vi "init subpanel.vi"(0 "References in":T2, 5 "Sub Panel":refnum<vi>, 7 "VI refnum":refnum<vi>, 9 "node ref":T1, 11 "error in (no error)":errorcluster) -> (15 "error IO":errorcluster)   [LabVIEW 2013, in "Scaling editor node.lvclass"]
uses:
  Scaling editor node.lvclass
  <vilib>/NI/DCAF Table API/Table Manager/references.ctl
  <vilib>/NI/Configuration Framework/Node/StopEvent.ctl
  <vilib>/NI/Configuration Framework/Node/RefreshUIEvent.ctl
  <vilib>/NI/Configuration Framework/Node/CacheState.ctl
  <vilib>/NI/Configuration Framework/Node/NodeChangeEvent.ctl
  <vilib>/NI/Configuration Framework/Node/NodeRef.ctl
  <vilib>/NI/Configuration Framework/Node/NISE_CEF_Node.lvclass
  <vilib>/NI/DCAF/Tag Editor Core/control module/editor node/channel action event.ctl
  <vilib>/NI/DCAF/Tag Editor Core/control module/editor node/dialog output action.ctl
  <vilib>/NI/Tag Bus Module Framework/channel/TBM channel.lvclass
  <vilib>/NI/Tag Bus/tag/tag descriptor.lvclass
  <vilib>/NI/AMC/Message Queue.ctl
  <vilib>/NI/AMC/Message.ctl
  <vilib>/NI/Tools/Keyed Array/KeyedArray.ctl
  <vilib>/NI/Configuration Framework/Node/UserEventRef.ctl
  <vilib>/NI/Configuration Framework/Controls/EventCluster.ctl
  <vilib>/NI/DCAF/Tag Editor Core/control module/editor node/control module editor.lvclass
  <vilib>/NI/Tools/Keyed Array/Tools_KeyedArray.lvlib
  <vilib>/NI/AMC/AMC.lvlib
  <vilib>/NI/Configuration Framework/NISE_CEF_TreeControl.lvlib
  <vilib>/NI/DCAF Table API/Table Manager/Table Manager.lvclass
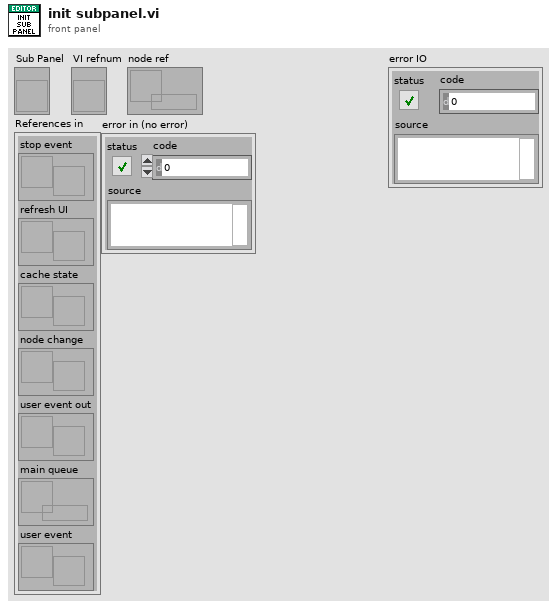
[diagram p1: front panel]
types:
  T1 = typedef "NISE_CEF_Node.lvclass/NodeRef.ctl" = refnum<data-value>
  T2 = typedef "Table Manager.lvlib/Table Manager.lvclass/references.ctl" = cluster{"stop event":T3, "refresh UI":T4, "cache state":T5, "node change":T6, "user event out":refnum<user-event>, "main queue":T7, "user event":T8}
  T3 = typedef "NISE_CEF_Node.lvclass/StopEvent.ctl" = refnum<user-event>
  T4 = typedef "NISE_CEF_Node.lvclass/RefreshUIEvent.ctl" = refnum<user-event>
  T5 = typedef "NISE_CEF_Node.lvclass/CacheState.ctl" = refnum<user-event>
  T6 = typedef "NISE_CEF_Node.lvclass/NodeChangeEvent.ctl" = refnum<user-event>
  T7 = typedef "AMC.lvlib/Message Queue.ctl" = refnum<queue>
  T8 = typedef "NISE_CEF_Node.lvclass/UserEventRef.ctl" = refnum<user-event>
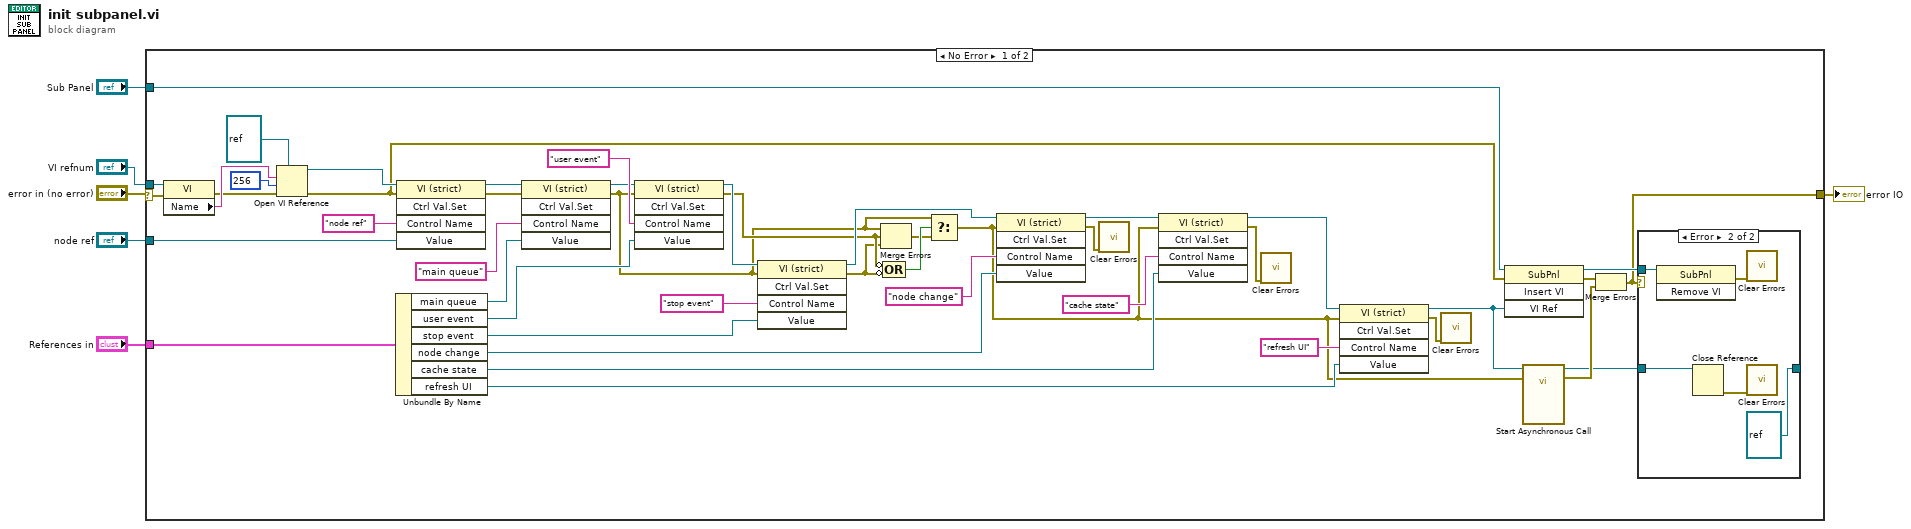
[diagram p0: block diagram]
diagram:
  n1 = case shown="No Error" "error in (no error)" {
    selector: "error in (no error)" -> [w8 w59]
    tunnel: "VI refnum" -> [w48 _]
    tunnel: "References in" -> [w44 _]
    tunnel: "Sub Panel" -> [w18 _]
    tunnel: "node ref" -> [w9 _]
    tunnel: [w7 w59] -> w1
    frame No Error {
      n2 = property class="VI"(reference=w48, error in=w8) -> (error out=w49:errorcluster, "Name"=w50:string)  [unwired: 1 out]
      n3 = Open VI Reference(type specifier VI Refnum (for type only)=refnum<vi> refnum, vi path=w50, options=256, error in (no error)=w49) -> (vi reference=w46:refnum<vi>, error out=w17:errorcluster)  [unwired: 2 in]
      n4 = Unbundle By Name(w44) -> ("main queue"=w32:T7, "user event"=w43:T8, "stop event"=w40:T3, "node change"=w38:T6, "cache state"=w23:T5, "refresh UI"=w19:T4)
      n5 = invoke class="VI (strict)" method="Ctrl Val.Set"(reference=w46, error in=w17, "Control Name"="node ref", "Value"=w9) -> (reference out=w34:refnum<vi>, error out=w33:errorcluster)  [unwired: 1 in, 3 out]
      n6 = invoke class="VI (strict)" method="Ctrl Val.Set"(reference=w34, error in=w33, "Control Name"="main queue", "Value"=w32) -> (reference out=w31:refnum<vi>, error out=w27:errorcluster)  [unwired: 1 in, 3 out]
      n7 = invoke class="VI (strict)" method="Ctrl Val.Set"(reference=w31, error in=w27, "Control Name"="user event", "Value"=w43) -> (reference out=w41:refnum<vi>, error out=w30:errorcluster)  [unwired: 1 in, 3 out]
      n8 = invoke class="VI (strict)" method="Ctrl Val.Set"(reference=w41, error in=w27, "Control Name"="stop event", "Value"=w40) -> (reference out=w37:refnum<vi>, error out=w29:errorcluster)  [unwired: 1 in, 3 out]
      n9 = Merge Errors(w27, w30, w29) -> (w28:errorcluster)
      n10 = Compound Arithmetic op=OR(invert w30, invert w29) -> (w36:bool)
      n11 = Select(t=w27, s=w36, f=w28) -> (s? t:f=w14:errorcluster)
      n12 = invoke class="VI (strict)" method="Ctrl Val.Set"(reference=w37, error in=w14, "Control Name"="node change", "Value"=w38) -> (reference out=w25:refnum<vi>, error out=w26:errorcluster)  [unwired: 1 in, 3 out]
      n13 = call <vilib>:"Clear Errors.vi"("error in (no error)"=w26) -> ()  [unwired: 6 in, 1 out]
      n14 = invoke class="VI (strict)" method="Ctrl Val.Set"(reference=w25, error in=w14, "Control Name"="cache state", "Value"=w23) -> (reference out=w21:refnum<vi>, error out=w22:errorcluster)  [unwired: 1 in, 3 out]
      n15 = call <vilib>:"Clear Errors.vi"("error in (no error)"=w22) -> ()  [unwired: 6 in, 1 out]
      n16 = invoke class="VI (strict)" method="Ctrl Val.Set"(reference=w21, error in=w14, "Control Name"="refresh UI", "Value"=w19) -> (reference out=w15:refnum<vi>, error out=w16:errorcluster)  [unwired: 1 in, 3 out]
      n17 = call <vilib>:"Clear Errors.vi"("error in (no error)"=w16) -> ()  [unwired: 6 in, 1 out]
      n18 = invoke class="SubPnl" method="Insert VI"(reference=w18, error in=w17, "VI Ref"=w15) -> (reference out=w11:refnum<vi>, error out=w13:errorcluster)  [unwired: 1 in, 2 out]
      n19 = call-by-ref "Start Asynchronous Call"(reference=w15, error in=w14) -> (reference out=w10:refnum<vi>, error out=w12:errorcluster)  [unwired: 12 in]
      n20 = Merge Errors(w13, w12) -> (w7:errorcluster)
      n21 = case shown="Error" w7 {
        tunnel: w10 -> [w53 w56]
        tunnel: [w53 refnum<vi> refnum ("type specifier VI Refnum (for type only)")] -> _
        tunnel: w11 -> [_ w54]
        frame No Error {
        }
        frame Error {
          n22 = invoke class="SubPnl" method="Remove VI"(reference=w54) -> (error out=w55:errorcluster)  [unwired: 2 in, 2 out]
          n23 = Close Reference(reference=w56) -> (error out=w58:errorcluster)  [unwired: 1 in]
          n24 = call <vilib>:"Clear Errors.vi"("error in (no error)"=w55) -> ()  [unwired: 6 in, 1 out]
          n25 = call <vilib>:"Clear Errors.vi"("error in (no error)"=w58) -> ()  [unwired: 6 in, 1 out]
        }
      }
    }
    frame Error {
    }
  }
  "error IO" <- w1
